vi "Variant To Type.vi"(7 "Required? (F)":bool, 10 "Type In":T1, 11 "Value":variant) -> (2 "Type":T1)   [LabVIEW 2020, in "FlexBlocks.lvlib"]
uses:
  FlexBlocks.lvlib
  Type Descriptor.ctl
  Terminal Direction.ctl
  Value Mode.ctl
  Special Terminal.ctl
  <vilib>/Utility/Data Type/NI_Data Type.lvlib
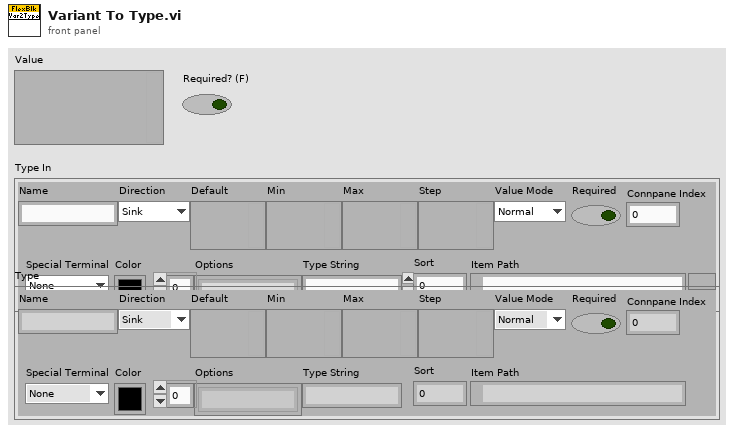
[diagram p1: front panel]
types:
  T1 = typedef "FlexBlocks.lvlib/Type Descriptor.ctl" = cluster{"Name":string, "Direction":T2, "Default":variant, "Min":variant, "Max":variant, "Step":variant, "Value Mode":T3, "Required":bool, "Connpane Index":i32, "Special Terminal":T4, "Color":u32, "Options":string[], "Type String":string, "Sort":i32, "Item Path":path}
  T2 = typedef "FlexBlocks.lvlib/Terminal Direction.ctl" = enum16{"Sink", "Source"}
  T3 = typedef "FlexBlocks.lvlib/Value Mode.ctl" = enum16{"Normal", "Range", "Select"}
  T4 = typedef "FlexBlocks.lvlib/Special Terminal.ctl" = enum16{"None", "Action", "Init", "Tag", "State in", "State out", "Error"}
  T5 = typedef "NI_Data Type.lvlib/Data Type.ctl" = enum8{"Invalid Type", "Void", "I8", "I16", "I32", "I64", "U8", "U16", "U32", "U64", "Single Float", "Double Float", "Extended Float", "Single Complex", "Double Complex", "Extended Complex", "Enum U8", "Enum U16", "Enum U32", "Enum U64", "Single Float With Unit", "Double Float With Unit", "Extended Float With Unit", "Single Complex with Unit", "Double Complex with Unit", "Extended Complex with Unit", "Boolean", "String", "Path", "Picture", "Tag", "Array", "Cluster", "Variant", "LV Variant", "Waveform", "Timestamp", "Digital Waveform", "Digital Data", "ExpressData", "Refnum", "External Data", "VI", "Poly VI", "LabVIEW Class Instance", "Fixed Point", "Set Collection", "Map Collection"}
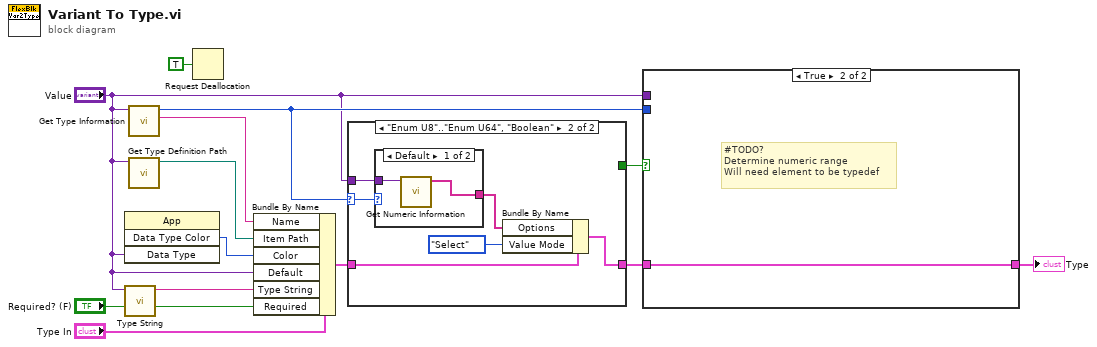
[diagram p0: block diagram]
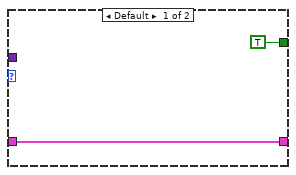
[diagram p3: hidden frame]
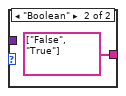
[diagram p4: hidden frame]
diagram:
  n1 = invoke class="App" method="Data Type Color"("Data Type"="Value") -> ("Data Type Color"=w11:u32)  [unwired: 3 in, 3 out]
  n2 = call "Type String.vi"("Type"="Value") -> ("Type String"=w4:string)  [unwired: 10 in]
  n3 = call <vilib>:"Get Type Information.vi"("variant"="Value") -> ("name"=w10:string, "type"=w7:T5)  [unwired: 6 in, 3 out]
  n4 = call <vilib>:"Get Type Definition Path.vi"("variant"="Value") -> ("type definition path"=w2:path)  [unwired: 9 in, 1 out]
  n5 = Request Deallocation(TRUE ("flag")) -> ()
  n6 = Bundle By Name(cluster="Type In", "Name"=w10, "Item Path"=w2, "Color"=w11, "Default"="Value", "Type String"=w4, "Required"="Required? (F)") -> (w9:T1)
  n7 = case shown="\"Enum U8\"..\"Enum U64\", \"Boolean\"" w7 {
    selector: w7 -> [_ w21]
    tunnel: w9 -> [w14 w19]
    tunnel: [TRUE _] -> w8
    tunnel: "Value" -> [_ w20]
    tunnel: [w14 w16] -> w6
    frame Default {
    }
    frame "Enum U8".."Enum U64", "Boolean" {
      n8 = case shown="Default" w21 {
        tunnel: w20 -> [w23 _]
        tunnel: [w22 string[] ["False", "True"]] -> w17
        frame Default {
          n9 = call <vilib>:"Get Numeric Information.vi"("variant"=w23) -> ("enum names"=w22:string[])  [unwired: 7 in, 3 out]
        }
        frame "Boolean" {
        }
      }
      n10 = Bundle By Name(cluster=w19, "Options"=w17, "Value Mode"=Value_Mode."Select") -> (w16:T1)
    }
  }
  n11 = case shown="True" w8 {
    tunnel: "Value" -> [_ _]
    tunnel: w7 -> [_ _]
    tunnel: w6 -> [w25 w26]
    tunnel: [w25 w26] -> w5
    frame False {
    }
    frame True {
      # "#TODO?\nDetermine numeric range\nWill need element to be typedef"
    }
  }
  "Type" <- w5
